vi "Write Return Address and Payload.vi"(7 "Reply Message":refnum<class "Message.lvclass">, 9 "Return Priority (Normal)":T1=enum."Normal", 10 "Return Address":refnum<class "Message Enqueuer.lvclass">, 11 "Dialog Return Msg in":refnum<class "Dialog Return Msg.lvclass">) -> (3 "Dialog Return Msg out":refnum<class "Dialog Return Msg.lvclass">)   [LabVIEW 2017, in "IDialogBox.lvlib" / "Dialog Return Msg.lvclass"]
doc: "<License>\nCopyright © 2017 Composed Systems, LLC | All rights reserved\nwww.composed.io\n\nAuthor: Ethan Stern <ethan.stern@composed.io>\n\nThis software is provided \"AS IS\" WITHOUT WARRANTIES, either express or implied, AND IS FOR EDUCATIONAL PURPOSES ONLY.\n</License>"
uses:
  Dialog Return Msg.lvclass
  C:/Git/mva-framework/Framework/AbstractMessages/PreAddressedMsg/PreAddressedMsg.lvclass
  <vilib>/ActorFramework/Message/Message.lvclass
  <vilib>/ActorFramework/Message Enqueuer/Message Enqueuer.lvclass
  <vilib>/ActorFramework/Message Enqueuer/Message Priority.ctl
  AbstractMessages/PreAddressedMsg/PreAddressedMsg.lvclass/PreAddressedMsg.ctl
  Dialog Return Msg.lvclass/Dialog Return Msg.ctl
  AbstractMessages/PreAddressedMsg/PreAddressedMsg.lvclass
panel:
  # "This input is here in case\nany future Actors want to\noverride the Dialog Return Msg.\nIf unwired, this method just\ninstantiates the basic message\ntype, which is good enough\nfor most reply scenarios."
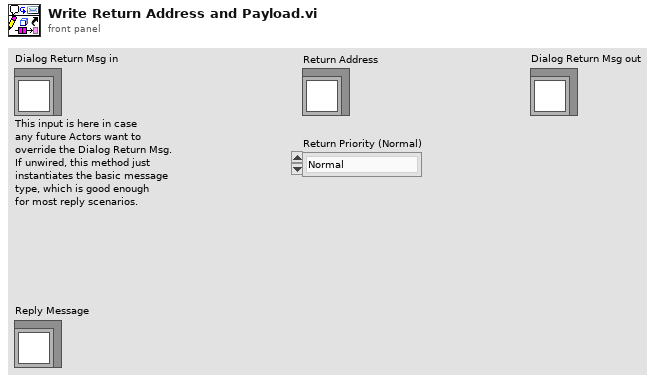
[diagram p1: front panel]
types:
  T1 = typedef "Actor Framework.lvlib/Message Enqueuer.lvclass/Message Priority.ctl" = enum16{"Low", "Normal", "High"}
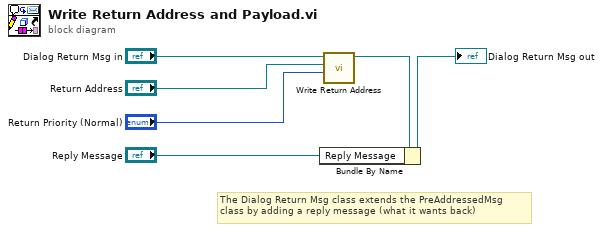
[diagram p0: block diagram]
diagram:
  # "The Dialog Return Msg class extends the PreAddressedMsg\nclass by adding a reply message (what it wants back)"
  n1 = call "Write Return Address.vi"("Return Priority (Normal)"="Return Priority (Normal)", "Return Address"="Return Address", "PreAddressedMsg in"="Dialog Return Msg in") -> ("PreAddressedMsg out"=w3:refnum<class "Dialog Return Msg.lvclass">)  [unwired: 8 in]
  n2 = Bundle By Name(cluster=w3, "Reply Message"="Reply Message") -> (→"Dialog Return Msg out":refnum<class "Dialog Return Msg.lvclass">)
